vi "AccelerometerTest.vi"() -> ()   [LabVIEW 2016]
uses:
  Telemetry/TelemetryFields.ctl
  <vilib>/rvi/Emulation/niFpgaGetClockAttributes.vi
  <vilib>/rvi/Emulation/niFpgaSctlEmulationGetInTimedLoop.vi
  <vilib>/rvi/Emulation/niFpgaEmulationReportErrorSimple.vi
  <vilib>/rvi/eio/common/nirviEmuTemplateMethod_errors.vi
  <vilib>/rvi/Emulation/niFpgaEmulationIsFPGAContextNoSignature.vi
  <vilib>/rvi/errors/niFpgaSetErrorForExecOnDevCompSimple.vi
  <vilib>/rvi/eio/common/nirviEmuReportErrorAndStop.vi
  <vilib>/rvi/DataTransferAndStorage/Container/Common/niFpgaContainerGetUniqueNameForEmu.vi
  <vilib>/rvi/FIFO/Fifo_Resource/nirvififoEmulationSetSize.vi
  <vilib>/rvi/FIFO/Fifo_Resource/nirviFifoEmulationQueueMgr.vi
  <instcachedir>/0/nirviFifoEmulationQueueMgr_E5CAEC123FF24DC58D834DCA3CDAA9B5.lvgen/nirviFifoEmulationQueueMgr_E5CAEC123FF24DC58D834DCA3CDAA9B5_004.vi
  <vilib>/rvi/FIFO/Fifo_Resource/nirvififoEmulationDetermineInputValidOut.vi
  <vilib>/rvi/FIFO/Fifo_Resource/nirvififoEmulationCreateLock.vi
  <vilib>/rvi/Emulation/niFpgaProcessEmulError.vi
  <vilib>/rvi/FIFO/Fifo_Resource/nirvififoEmulationObtainLock.vi
  <vilib>/rvi/FIFO/Fifo_Resource/nirvififoEmulationReleaseLock.vi
  <vilib>/rvi/occurrence/nirviWaitOnOccurrenceBase.vi
  <vilib>/rvi/errors/nirviReportUnexpectedCaseInternalError.vi
  <vilib>/rvi/errors/nirviReportUnexpectedCaseInternalError (U32).vi
  <vilib>/Utility/error.llb/Clear Errors.vi
  <vilib>/rvi/Emulation/niFpgaCriticalErrorInLSC.vi
  <vilib>/eio/EIONode/EIONode.xnode
  <vilib>/rvi/DataTransferAndStorage/Container/XNode/niFpgaContainer.xnode
  <vilib>/rvi/FIFO/Fifo_Resource/nirvififoEmulationWrite.vi
  <vilib>/rvi/FIFO/Fifo_Resource/nirvififoEmulationRead.vi
panel:
  out "Time":u64
  out "AngularAccelerationZ":sgl format="%#.6f"
  out "AngularAccelerationY":sgl format="%#.6f"
  out "AngularAccelerationX":sgl format="%#.6f"
  out "AccelerometerEng8":sgl format="%#.6f"
  out "AccelerometerEng7":sgl format="%#.6f"
  out "AccelerometerEng6":sgl format="%#.6f"
  out "AccelerometerEng5":sgl format="%#.6f"
  out "AccelerometerEng4":sgl format="%#.6f"
  out "AccelerometerEng3":sgl format="%#.6f"
  out "AccelerometerEng2":sgl format="%#.6f"
  out "AccelerometerEng1":sgl format="%#.6f"
  out "AccelerometerTimestamp":u64
  out "AccelerometerRaw1":sgl format="%#.6f"
  out "AccelerometerRaw2":sgl format="%#.6f"
  out "AccelerometerRaw3":sgl format="%#.6f"
  out "AccelerometerRaw4":sgl format="%#.6f"
  out "AccelerometerRaw5":sgl format="%#.6f"
  out "AccelerometerRaw6":sgl format="%#.6f"
  out "AccelerometerRaw7":sgl format="%#.6f"
  out "AccelerometerRaw8":sgl format="%#.6f"
  out "AccelerometerSampleCount":u64
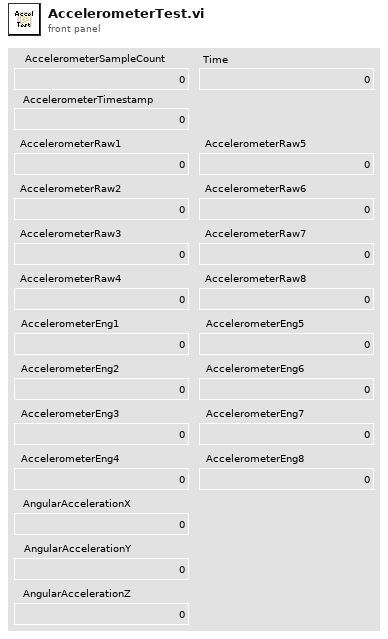
[diagram p1: front panel]
types:
  T1 = typedef "TelemetryFields.ctl" = enum16{"InclinometerErrorCode", "InclinometerTxBytes", "InclinometerRxBytes", "InclinometerTxFrames", "InclinometerRxFrames", "InclinometerTimestamp", "InclinometerAngle", "DisplacementErrorCode", "DisplacementTxBytes", "DisplacementRxBytes", "DisplacementTxFrames", "DisplacementRxFrames", "DisplacementTimestamp", "Displacement1", "Displacement2", "Displacement3", "Displacement4", "Displacement5", "Displacement6", "Displacement7", "Displacement8", "AccelerometerSampleCount", "AccelerometerTimestamp", "AccelerometerRaw1", "AccelerometerRaw2", "AccelerometerRaw3", "AccelerometerRaw4", "AccelerometerRaw5", "AccelerometerRaw6", "AccelerometerRaw7", "AccelerometerRaw8", "AccelerometerEng1", "AccelerometerEng2", "AccelerometerEng3", "AccelerometerEng4", "AccelerometerEng5", "AccelerometerEng6", "AccelerometerEng7", "AccelerometerEng8", "AngularAccelerationX", "AngularAccelerationY", "AngularAccelerationZ"}
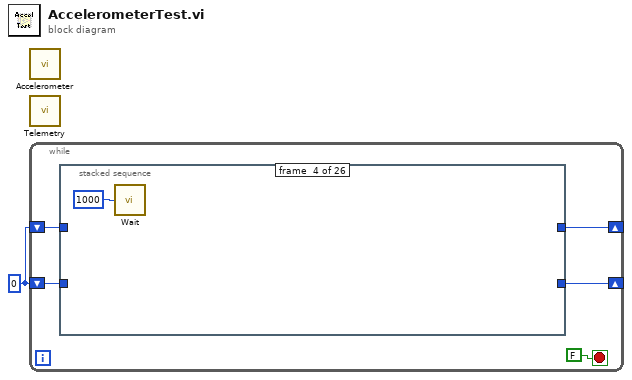
[diagram p0: block diagram]
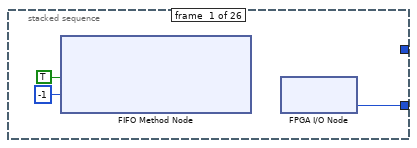
[diagram p2: hidden frame]
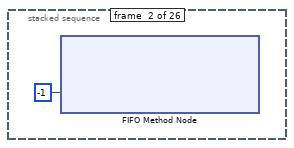
[diagram p3: hidden frame]
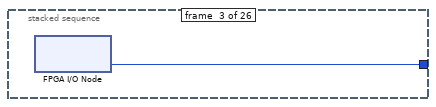
[diagram p4: hidden frame]
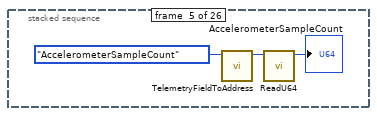
[diagram p5: hidden frame]
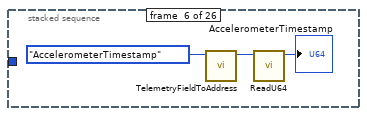
[diagram p6: hidden frame]
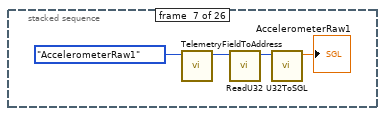
[diagram p7: hidden frame]
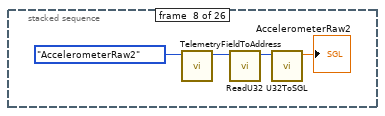
[diagram p8: hidden frame]
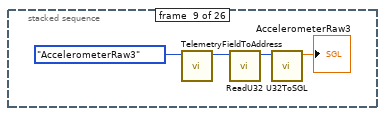
[diagram p9: hidden frame]
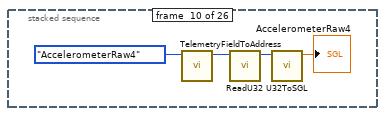
[diagram p10: hidden frame]
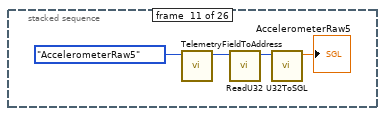
[diagram p11: hidden frame]
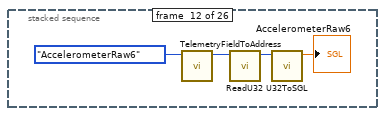
[diagram p12: hidden frame]
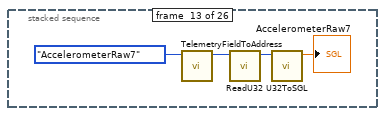
[diagram p13: hidden frame]
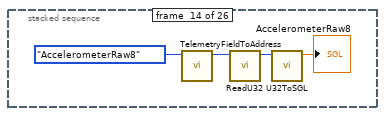
[diagram p14: hidden frame]
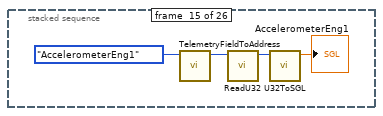
[diagram p15: hidden frame]
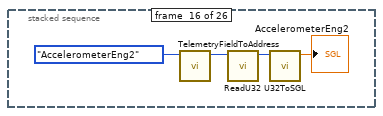
[diagram p16: hidden frame]
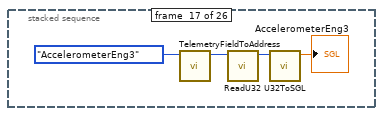
[diagram p17: hidden frame]
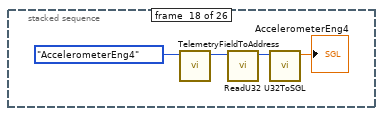
[diagram p18: hidden frame]
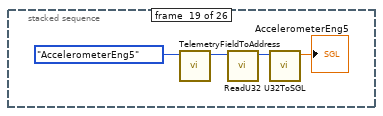
[diagram p19: hidden frame]
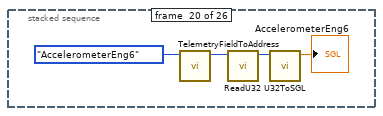
[diagram p20: hidden frame]
diagram:
  w1 = u64 0 ("Time")
  n1 = call "Accelerometer.vi"() -> ()  [unwired: 12 in]
  n2 = call "Telemetry.vi"() -> ()  [unwired: 12 in]
  n3 = while {
    shift-right: [w5] -> _
    shift-left: w1 -> [w4]
    shift-right: [w3] -> _
    shift-left: w1 -> [w2]
    stop <- FALSE stop-if-true
    n4 = stacked-sequence {
      tunnel: [w9 _ _ _ _ _ _ _ _ _ _ _ _ _ _ _ _ _ _ _ _ _ _ _ _ _] -> w5
      tunnel: w4 -> [_ _ _ _ _ _ _ _ _ _ _ _ _ _ _ _ _ _ _ _ _ _ _ _ _ w97]
      tunnel: [_ _ w11 _ _ _ _ _ _ _ _ _ _ _ _ _ _ _ _ _ _ _ _ _ _ _] -> w3
      tunnel: w2 -> [_ _ _ _ _ _ _ _ _ _ _ _ _ _ _ _ _ _ _ _ _ _ _ _ _ w95]
      frame #0 {
        n5 = xnode ("FIFO Method Node")("Element"=TRUE, "Timeout"=-1) -> ()  [unwired: 1 in, 2 out]
        n6 = xnode "FPGA I/O Node"() -> ("Time"=w9:u64)  [unwired: 1 in, 1 out]
      }
      frame #1 {
        n7 = xnode ("FIFO Method Node")("Timeout"=-1) -> ()  [unwired: 1 in, 3 out]
      }
      frame #2 {
        n8 = xnode "FPGA I/O Node"() -> ("Time"=w11:u64)  [unwired: 1 in, 1 out]
      }
      frame #3 {
        n9 = call "Wait"("Count(uSec)"=u32 1000 ("Count(mSec)")) -> ()  [unwired: 1 out]
      }
      frame #4 {
        n10 = call "TelemetryFieldToAddress.vi"("TelemetryFields"=TelemetryFields."AccelerometerSampleCount") -> ("Address"=w14:u32)  [unwired: 10 in]
        n11 = call "ReadU64.vi"("Address"=w14) -> ("Data"=→"AccelerometerSampleCount":u64)  [unwired: 10 in]
      }
      frame #5 {
        n12 = call "TelemetryFieldToAddress.vi"("TelemetryFields"=TelemetryFields."AccelerometerTimestamp") -> ("Address"=w18:u32)  [unwired: 10 in]
        n13 = call "ReadU64.vi"("Address"=w18) -> ("Data"=→"AccelerometerTimestamp":u64)  [unwired: 10 in]
      }
      frame #6 {
        n14 = call "TelemetryFieldToAddress.vi"("TelemetryFields"=TelemetryFields."AccelerometerRaw1") -> ("Address"=w22:u32)  [unwired: 10 in]
        n15 = call "ReadU32.vi"("Address"=w22) -> ("Data"=w21:u32)  [unwired: 10 in]
        n16 = call "U32ToSGL.vi"("U32"=w21) -> ("SGL"=→"AccelerometerRaw1":sgl)  [unwired: 10 in]
      }
      frame #7 {
        n17 = call "TelemetryFieldToAddress.vi"("TelemetryFields"=TelemetryFields."AccelerometerRaw2") -> ("Address"=w26:u32)  [unwired: 10 in]
        n18 = call "ReadU32.vi"("Address"=w26) -> ("Data"=w25:u32)  [unwired: 10 in]
        n19 = call "U32ToSGL.vi"("U32"=w25) -> ("SGL"=→"AccelerometerRaw2":sgl)  [unwired: 10 in]
      }
      frame #8 {
        n20 = call "TelemetryFieldToAddress.vi"("TelemetryFields"=TelemetryFields."AccelerometerRaw3") -> ("Address"=w30:u32)  [unwired: 10 in]
        n21 = call "ReadU32.vi"("Address"=w30) -> ("Data"=w29:u32)  [unwired: 10 in]
        n22 = call "U32ToSGL.vi"("U32"=w29) -> ("SGL"=→"AccelerometerRaw3":sgl)  [unwired: 10 in]
      }
      frame #9 {
        n23 = call "TelemetryFieldToAddress.vi"("TelemetryFields"=TelemetryFields."AccelerometerRaw4") -> ("Address"=w34:u32)  [unwired: 10 in]
        n24 = call "ReadU32.vi"("Address"=w34) -> ("Data"=w33:u32)  [unwired: 10 in]
        n25 = call "U32ToSGL.vi"("U32"=w33) -> ("SGL"=→"AccelerometerRaw4":sgl)  [unwired: 10 in]
      }
      frame #10 {
        n26 = call "TelemetryFieldToAddress.vi"("TelemetryFields"=TelemetryFields."AccelerometerRaw5") -> ("Address"=w38:u32)  [unwired: 10 in]
        n27 = call "ReadU32.vi"("Address"=w38) -> ("Data"=w37:u32)  [unwired: 10 in]
        n28 = call "U32ToSGL.vi"("U32"=w37) -> ("SGL"=→"AccelerometerRaw5":sgl)  [unwired: 10 in]
      }
      frame #11 {
        n29 = call "TelemetryFieldToAddress.vi"("TelemetryFields"=TelemetryFields."AccelerometerRaw6") -> ("Address"=w42:u32)  [unwired: 10 in]
        n30 = call "ReadU32.vi"("Address"=w42) -> ("Data"=w41:u32)  [unwired: 10 in]
        n31 = call "U32ToSGL.vi"("U32"=w41) -> ("SGL"=→"AccelerometerRaw6":sgl)  [unwired: 10 in]
      }
      frame #12 {
        n32 = call "TelemetryFieldToAddress.vi"("TelemetryFields"=TelemetryFields."AccelerometerRaw7") -> ("Address"=w46:u32)  [unwired: 10 in]
        n33 = call "ReadU32.vi"("Address"=w46) -> ("Data"=w45:u32)  [unwired: 10 in]
        n34 = call "U32ToSGL.vi"("U32"=w45) -> ("SGL"=→"AccelerometerRaw7":sgl)  [unwired: 10 in]
      }
      frame #13 {
        n35 = call "TelemetryFieldToAddress.vi"("TelemetryFields"=TelemetryFields."AccelerometerRaw8") -> ("Address"=w50:u32)  [unwired: 10 in]
        n36 = call "ReadU32.vi"("Address"=w50) -> ("Data"=w49:u32)  [unwired: 10 in]
        n37 = call "U32ToSGL.vi"("U32"=w49) -> ("SGL"=→"AccelerometerRaw8":sgl)  [unwired: 10 in]
      }
      frame #14 {
        n38 = call "TelemetryFieldToAddress.vi"("TelemetryFields"=TelemetryFields."AccelerometerEng1") -> ("Address"=w54:u32)  [unwired: 10 in]
        n39 = call "ReadU32.vi"("Address"=w54) -> ("Data"=w53:u32)  [unwired: 10 in]
        n40 = call "U32ToSGL.vi"("U32"=w53) -> ("SGL"=→"AccelerometerEng1":sgl)  [unwired: 10 in]
      }
      frame #15 {
        n41 = call "TelemetryFieldToAddress.vi"("TelemetryFields"=TelemetryFields."AccelerometerEng2") -> ("Address"=w58:u32)  [unwired: 10 in]
        n42 = call "ReadU32.vi"("Address"=w58) -> ("Data"=w57:u32)  [unwired: 10 in]
        n43 = call "U32ToSGL.vi"("U32"=w57) -> ("SGL"=→"AccelerometerEng2":sgl)  [unwired: 10 in]
      }
      frame #16 {
        n44 = call "TelemetryFieldToAddress.vi"("TelemetryFields"=TelemetryFields."AccelerometerEng3") -> ("Address"=w62:u32)  [unwired: 10 in]
        n45 = call "ReadU32.vi"("Address"=w62) -> ("Data"=w61:u32)  [unwired: 10 in]
        n46 = call "U32ToSGL.vi"("U32"=w61) -> ("SGL"=→"AccelerometerEng3":sgl)  [unwired: 10 in]
      }
      frame #17 {
        n47 = call "TelemetryFieldToAddress.vi"("TelemetryFields"=TelemetryFields."AccelerometerEng4") -> ("Address"=w66:u32)  [unwired: 10 in]
        n48 = call "ReadU32.vi"("Address"=w66) -> ("Data"=w65:u32)  [unwired: 10 in]
        n49 = call "U32ToSGL.vi"("U32"=w65) -> ("SGL"=→"AccelerometerEng4":sgl)  [unwired: 10 in]
      }
      frame #18 {
        n50 = call "TelemetryFieldToAddress.vi"("TelemetryFields"=TelemetryFields."AccelerometerEng5") -> ("Address"=w70:u32)  [unwired: 10 in]
        n51 = call "ReadU32.vi"("Address"=w70) -> ("Data"=w69:u32)  [unwired: 10 in]
        n52 = call "U32ToSGL.vi"("U32"=w69) -> ("SGL"=→"AccelerometerEng5":sgl)  [unwired: 10 in]
      }
      frame #19 {
        n53 = call "TelemetryFieldToAddress.vi"("TelemetryFields"=TelemetryFields."AccelerometerEng6") -> ("Address"=w74:u32)  [unwired: 10 in]
        n54 = call "ReadU32.vi"("Address"=w74) -> ("Data"=w73:u32)  [unwired: 10 in]
        n55 = call "U32ToSGL.vi"("U32"=w73) -> ("SGL"=→"AccelerometerEng6":sgl)  [unwired: 10 in]
      }
      frame #20 {
        n56 = call "TelemetryFieldToAddress.vi"("TelemetryFields"=TelemetryFields."AccelerometerEng7") -> ("Address"=w78:u32)  [unwired: 10 in]
        n57 = call "ReadU32.vi"("Address"=w78) -> ("Data"=w77:u32)  [unwired: 10 in]
        n58 = call "U32ToSGL.vi"("U32"=w77) -> ("SGL"=→"AccelerometerEng7":sgl)  [unwired: 10 in]
      }
      frame #21 {
        n59 = call "TelemetryFieldToAddress.vi"("TelemetryFields"=TelemetryFields."AccelerometerEng8") -> ("Address"=w82:u32)  [unwired: 10 in]
        n60 = call "ReadU32.vi"("Address"=w82) -> ("Data"=w81:u32)  [unwired: 10 in]
        n61 = call "U32ToSGL.vi"("U32"=w81) -> ("SGL"=→"AccelerometerEng8":sgl)  [unwired: 10 in]
      }
      frame #22 {
        n62 = call "TelemetryFieldToAddress.vi"("TelemetryFields"=TelemetryFields."AngularAccelerationX") -> ("Address"=w86:u32)  [unwired: 10 in]
        n63 = call "ReadU32.vi"("Address"=w86) -> ("Data"=w85:u32)  [unwired: 10 in]
        n64 = call "U32ToSGL.vi"("U32"=w85) -> ("SGL"=→"AngularAccelerationX":sgl)  [unwired: 10 in]
      }
      frame #23 {
        n65 = call "TelemetryFieldToAddress.vi"("TelemetryFields"=TelemetryFields."AngularAccelerationY") -> ("Address"=w90:u32)  [unwired: 10 in]
        n66 = call "ReadU32.vi"("Address"=w90) -> ("Data"=w89:u32)  [unwired: 10 in]
        n67 = call "U32ToSGL.vi"("U32"=w89) -> ("SGL"=→"AngularAccelerationY":sgl)  [unwired: 10 in]
      }
      frame #24 {
        n68 = call "TelemetryFieldToAddress.vi"("TelemetryFields"=TelemetryFields."AngularAccelerationZ") -> ("Address"=w94:u32)  [unwired: 10 in]
        n69 = call "ReadU32.vi"("Address"=w94) -> ("Data"=w93:u32)  [unwired: 10 in]
        n70 = call "U32ToSGL.vi"("U32"=w93) -> ("SGL"=→"AngularAccelerationZ":sgl)  [unwired: 10 in]
      }
      frame #25 {
        n71 = Subtract(x=w95, y=w97) -> (x-y=→"Time":u64)
      }
    }
  }
